vi "Write Thermocouple Type.vi"(8 "error in (no error)":errorcluster, 10 "Thermocouple Type":T1, 11 "Thermocouple in":refnum<class "Thermocouple.lvclass">) -> (0 "error out":errorcluster, 3 "Thermocouple out":refnum<class "Thermocouple.lvclass">)   [LabVIEW 2018, in "Thermocouple.lvlib" / "Thermocouple.lvclass"]
uses:
  Thermocouple.lvclass
  Custom Controls/Thermocouple Type.ctl
  Thermocouple.lvclass/Thermocouple.ctl
  Thermocouple.lvlib
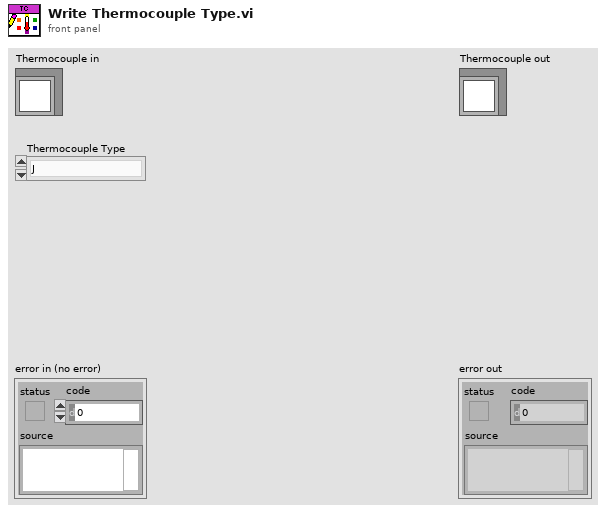
[diagram p1: front panel]
types:
  T1 = typedef "Thermocouple.lvlib/Thermocouple Type.ctl" = enum16{"J", "K", "N", "R", "S", "T", "B", "E"}
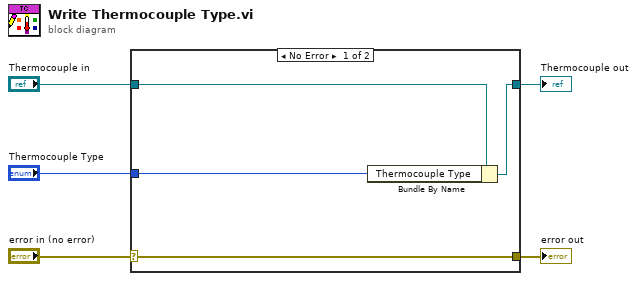
[diagram p0: block diagram]
diagram:
  n1 = case shown="No Error" "error in (no error)" {
    selector: "error in (no error)" -> [w9 w10]
    tunnel: [w9 w10] -> w4
    tunnel: [w7 w11] -> w2
    tunnel: "Thermocouple in" -> [w8 w11]
    tunnel: "Thermocouple Type" -> [w6 _]
    frame No Error {
      n2 = Bundle By Name(cluster=w8, "Thermocouple Type"=w6) -> (w7:refnum<class "Thermocouple.lvclass">)
    }
    frame Error {
    }
  }
  "error out" <- w4
  "Thermocouple out" <- w2
